vi "CONVERTIDOR.vi"() -> ()   [LabVIEW 2016]
panel:
  in  "stop":bool
  out "FAHRENHEIT":dbl
  in  "CENTIGRADOS":dbl
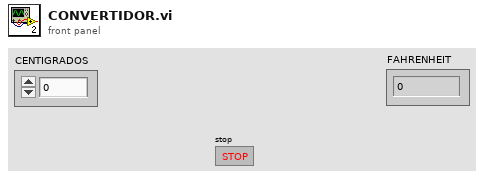
[diagram p1: front panel]
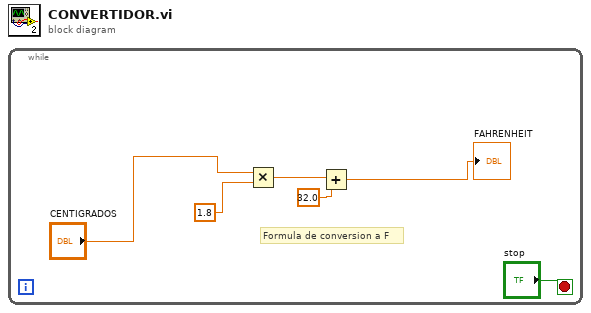
[diagram p0: block diagram]
diagram:
  n1 = while {
    stop <- "stop" stop-if-true
    # "Formula de conversion a F"
    n2 = Multiply(x="CENTIGRADOS", y=1.8) -> (x*y=w6:dbl)
    n3 = Add(x=w6, y=32.0) -> (x+y=→"FAHRENHEIT":dbl)
  }
